vi "LVClass_CorrectionDataManager ComputeDeltaCmdFromDeltaSWithCLSmooth.vi"(0 "CorrectionDataManager in":refnum<class "CorrectionDataManager.lvclass">, 5 "Delta Slopes IN":refnum<class "HasoSlopes.lvclass">, 7 "Gain in":dbl min=0.0 max=1.0, 9 "ClosedLoopSmoothing in":refnum<class "ClosedLoopSmoothing.lvclass">, 11 "error in (no error)":errorcluster, 12 "do tilt check":bool=TRUE) -> (4 "CorrectionDataManager out":refnum<class "CorrectionDataManager.lvclass">, 6 "Delta Slopes OUT":refnum<class "HasoSlopes.lvclass">, 8 "Gain out":dbl min=0.0 max=1.0, 10 "ClosedLoopSmoothing out":refnum<class "ClosedLoopSmoothing.lvclass">, 13 "DeltaPosition":T1, 15 "error out":errorcluster)   [LabVIEW 2020, in "CorrectionDataManager.lvclass"]
doc: "Compute the commands associated to one closed-loop iteration targeting\ndelta_slopes.\n\n<B>corrdata_managerIn</B> : CorrDataManager object.\n<B>corrdata_managerOut</B> : CorrDataManager object.\n<B>delta_slopes</B> : Array of target slopes deltas (stored as HasoSlopes).\n<B>delta_command</B> : Array of size actuators count, containing the commands deltas (relatives\n variations to apply from actuators initial positions).\n<B>do_tilt_check</B> : Indicates if the computed commands deltas must be adapted to avoid huge tilts.\n<B>smoothing_params</B> : Closed Loop smoothing params object.\n<B>specified_loop_gain</B> : User specified loop smoothing gain\n<B>applied_loop_gain</B> : Loop smoothing gain really applied"
uses:
  CorrectionDataManager.lvclass
  HasoSlopes.lvclass
  Wavefront Corrector Position.ctl
  ClosedLoopSmoothing.lvclass
  CorrectionDataManager.lvclass/CorrectionDataManager.ctl
  LVClass_ClosedLoopSmoothing Read ClosedLoopSmooth.vi
  LVClass_HasoSlopes Read HasoSlopes _ property.vi
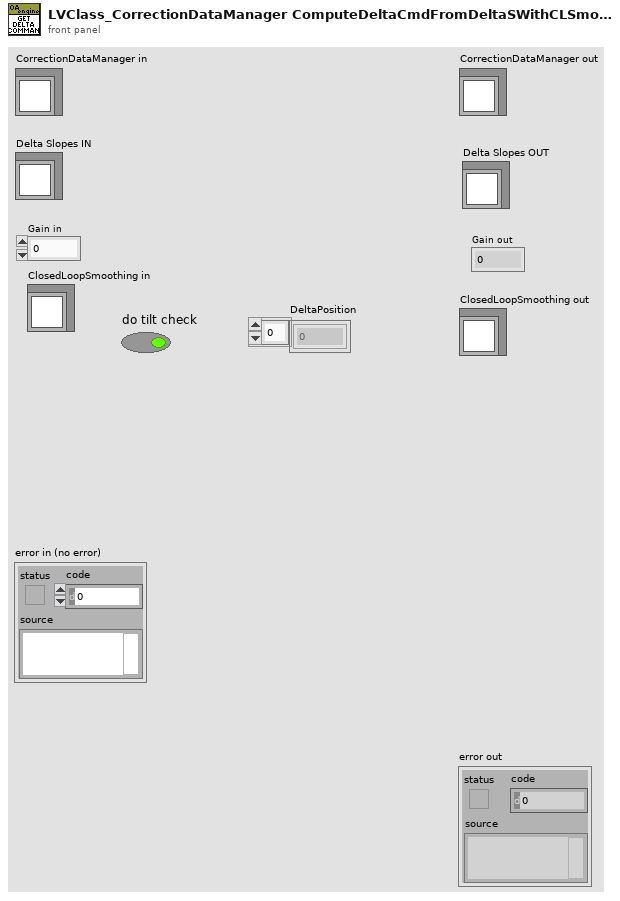
[diagram p1: front panel]
types:
  T1 = typedef "Wavefront Corrector Position.ctl" = sgl[]
  T2 = typedef "Wavefront Corrector states - ONE.ctl" = cluster{"Max":sgl, "Min":sgl, "Validity":enum16{"valid", "fixed", "invalid"}, "Fixed_Position":sgl}
  T3 = typedef "ClassID.ctl" = i64
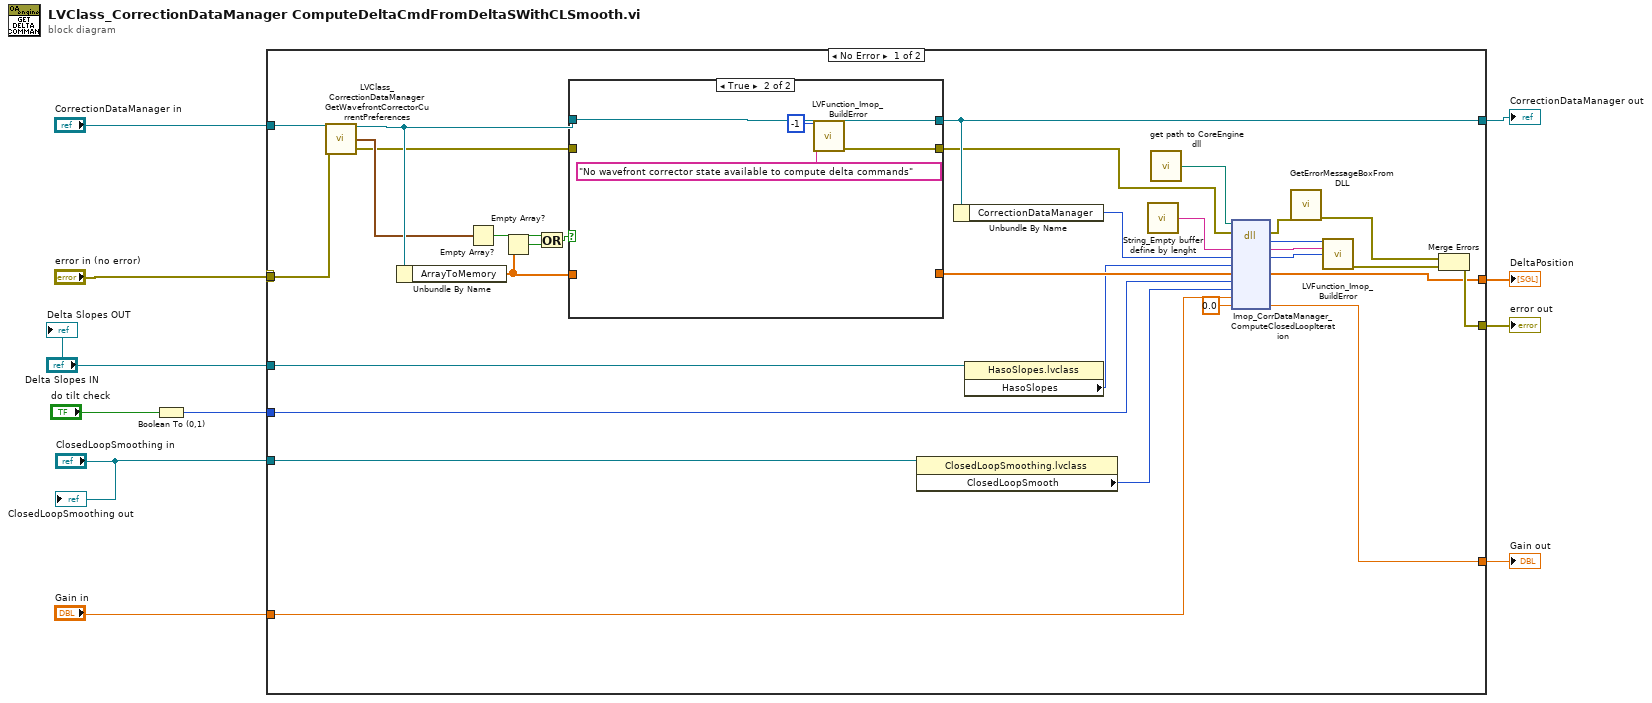
[diagram p0: block diagram]
diagram:
  n1 = Boolean To (0,1)(Boolean="do tilt check") -> (0, 1=w2:i16)
  n2 = case shown="No Error" "error in (no error)" {
    selector: "error in (no error)" -> [_ w51]
    tunnel: [w35 w51] -> w11
    tunnel: [w16 w50] -> w10
    tunnel: "CorrectionDataManager in" -> [w26 w50]
    tunnel: "Delta Slopes IN" -> [w19 _]
    tunnel: "Gain in" -> [w34 _]
    tunnel: [w33 _] -> w6
    tunnel: "ClosedLoopSmoothing in" -> [w21 _]
    tunnel: [w20 _] -> w4
    tunnel: w2 -> [w17 _]
    tunnel: "error in (no error)" -> [w13 _]
    frame No Error {
      n3 = call "LVClass_CorrectionDataManager GetWavefrontCorrectorCurrentPreferences.vi"("CorrectionDataManager in"=w26, "error in (no error)"=w13) -> ("CorrectionDataManager out"=w25:refnum<class "CorrectionDataManager.lvclass">, "Wavefront Corrector State"=w24:T2[], "error out"=w14:errorcluster)  [unwired: 11 in]
      n4 = Unbundle By Name(w25) -> ("ArrayToMemory"=w27:T1)
      n5 = Empty Array?(array=w24) -> (empty?=w30:bool)
      n6 = Empty Array?(array=w27) -> (empty?=w31:bool)
      n7 = Or(x=w31, y=w30) -> (x .or. y?=w29:bool)
      n8 = case shown="True" w29 {
        tunnel: w25 -> [w44 w49]
        tunnel: [w44 w49] -> w16
        tunnel: [w43 w48] -> w15
        tunnel: [w45 _] -> w28
        tunnel: w27 -> [w45 _]
        tunnel: w14 -> [w43 _]
        frame False {
        }
        frame True {
          n9 = call "LVFunction_Imop_BuildError.vi"("code"=-1, "String to Prepend to source (\"\")"="No wavefront corrector state available to compute delta commands" ("String to Prepend to source (\"\")")) -> ("error out"=w48:errorcluster)  [unwired: 13 in]
        }
      }
      n10 = property class="ClosedLoopSmoothing.lvclass"(reference=w21) -> ("ClosedLoopSmooth"=w22:T3)  [unwired: 1 in, 2 out]
      n11 = Unbundle By Name(w16) -> ("CorrectionDataManager"=w32:T3)
      n12 = property class="HasoSlopes.lvclass"(reference=w19) -> ("HasoSlopes"=w18:T3)  [unwired: 1 in, 2 out]
      n13 = call "String_Empty buffer define by lenght.vi"() -> ("Empty buffer"=w40:string)  [unwired: 1 in]
      n14 = call "get path to CoreEngine dll.vi"() -> ("path to wavekit library"=w39:path)  [unwired: 14 in, 1 out]
      n15 = dll-call lib="D:/FLE/0.Code/CoreEngine4_Suite/LV2011_interface/DLLs/c_interface_vc100.dll" fn="Imop_CorrDataManager_ComputeClosedLoopIteration"(path in=w39, error in=w15, "message"=w40, "WavefrontCorrection"=w32, "deltaHasoSlopes"=w18, "delta_commands"=w28, "do tilt check"=w17, "smoothing_params"=w22, "specified_loop_gain"=w34, "applied_loop_gain"=sgl 0.0) -> (error out=w38:errorcluster, "return type"=w42:i32, "message"=w41:string, "WavefrontCorrection"=w12:i64, "delta_commands"=w33:sgl[], "applied_loop_gain"=w20:sgl)  [unwired: 5 in, 1 out]
      n16 = call "GetErrorMessageBoxFromDLL.vi"("error IN"=w38) -> ("error OUT"=w37:errorcluster)  [unwired: 10 in]
      n17 = call "LVFunction_Imop_BuildError.vi"("code"=w42, "String to Prepend to source (\"\")"=w41, "Adresse"=w12) -> ("error out"=w36:errorcluster)  [unwired: 12 in]
      n18 = Merge Errors(w37, w36) -> (w35:errorcluster)
    }
    frame Error {
    }
  }
  "error out" <- w11
  "CorrectionDataManager out" <- w10
  "DeltaPosition" <- w6
  "Gain out" <- w4
  "Delta Slopes OUT" <- "Delta Slopes IN"
  "ClosedLoopSmoothing out" <- "ClosedLoopSmoothing in"
